vi "DetermineSpeedCap.vi"(2 "Speed Cap Decceleration Limit (ft/s^2)":dbl=15.0, 3 "Driver Profile Doesn't Want to Shift":bool) -> (0 "Speed Cap [0,1]":dbl)   [LabVIEW 2020]
doc: "Determines the speed cap for the swerve drive based on the control inputs and master alarms. This includes forcing the robot into low gear."
uses:
  GlobalDriverStationCommands.vi
  GlobalDrivebase.vi
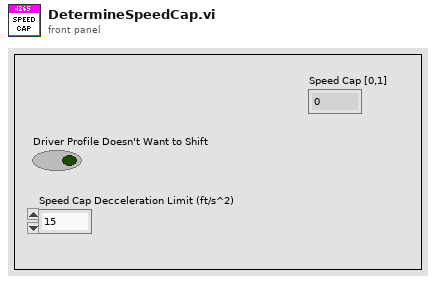
[diagram p1: front panel]
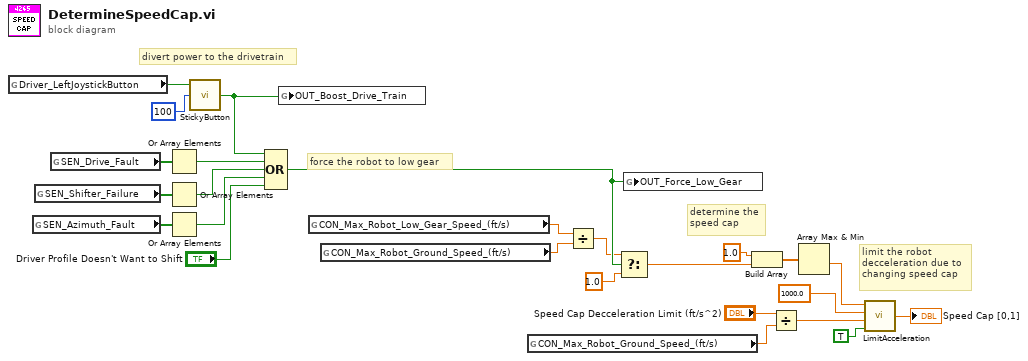
[diagram p0: block diagram]
diagram:
  # "limit the robot\ndecceleration due to\nchanging speed cap"
  # "force the robot to low gear"
  # "determine the\nspeed cap"
  # "divert power to the drivetrain"
  n1 = global read "GlobalDriverStationCommands.vi" "Driver_LeftJoystickButton"() -> (w7:bool)
  n2 = global read "GlobalDrivebase.vi" "SEN_Azimuth_Fault"() -> (w24:bool[])
  n3 = global read "GlobalDrivebase.vi" "SEN_Shifter_Failure"() -> (w25:bool[])
  n4 = global read "GlobalDrivebase.vi" "SEN_Drive_Fault"() -> (w3:bool[])
  n5 = Or Array Elements(Boolean array=w3) -> (logical OR=w2:bool)
  n6 = Or Array Elements(Boolean array=w25) -> (logical OR=w11:bool)
  n7 = Or Array Elements(Boolean array=w24) -> (logical OR=w10:bool)
  n8 = call "StickyButton.vi"("Time threshold (ms)"=u32 100 ("y"), "Button Input"=w7) -> ("Sticky Button"=w1:bool)  [unwired: 1 in]
  n9 = Compound Arithmetic op=OR(w1, w2, w11, w10, "Driver Profile Doesn't Want to Shift") -> (w23:bool)
  n10 = global write "GlobalDrivebase.vi" "OUT_Boost_Drive_Train"(w1) -> ()
  n11 = global read "GlobalDrivebase.vi" "CON_Max_Robot_Low_Gear_Speed_(ft/s)"() -> (w21:dbl)
  n12 = global read "GlobalDrivebase.vi" "CON_Max_Robot_Ground_Speed_(ft/s)"() -> (w22:dbl)
  n13 = global read "GlobalDrivebase.vi" "CON_Max_Robot_Ground_Speed_(ft/s)"() -> (w5:dbl)
  n14 = Divide(x=w21, y=w22) -> (x/y=w18:dbl)
  n15 = Select(t=w18, s=w23, f=1.0) -> (s? t:f=w19:dbl)
  n16 = global write "GlobalDrivebase.vi" "OUT_Force_Low_Gear"(w23) -> ()
  n17 = Build Array(1.0 ("element"), w19) -> (w12:dbl[])
  n18 = Divide(x="Speed Cap Decceleration Limit (ft/s^2)", y=w5) -> (x/y=w4:dbl)
  n19 = Array Max & Min(array=w12) -> (min value=w15:dbl)  [unwired: 3 out]
  n20 = call "LimitAcceleration.vi"("Apply Limit"=TRUE, "Decceleration Limit (/s)"=w4, "Acceleration Limit (/s)"=1000.0, "Raw Input"=w15) -> ("Output"=→"Speed Cap [0,1]":dbl)
